vi "ColourBandPicker.vi"() -> ()   [LabVIEW 2021]
uses:
  <vilib>/userDefined/High Color/IMAQdx.ctl
  <vilib>/vision/driver/IMAQdx.llb/IMAQdx Camera Control Mode.ctl
  <vilib>/vision/driver/IMAQdx.llb/IMAQdx Acquisition Mode.ctl
  <vilib>/vision/driver/IMAQdx.llb/IMAQdx Buffer Number Mode.ctl
  <vilib>/vision/driver/NI_Vision_Acquisition_Software.lvlib
  <resource>/objmgr/imaqdx.rc
  <vilib>/vision/NI_Vision_Development_Module.lvlib
panel:
  out "Color Box":u32(colorbox)
  out "Colour Value":u32
  out "Model":string
  out "Attr":T1(array[cluster]) caption="Camera Attributes"
  out "Image":T2(plugin-control)
  in  "Stop":bool
  out "error out":errorcluster
  # "RPV Test Rig 2024"
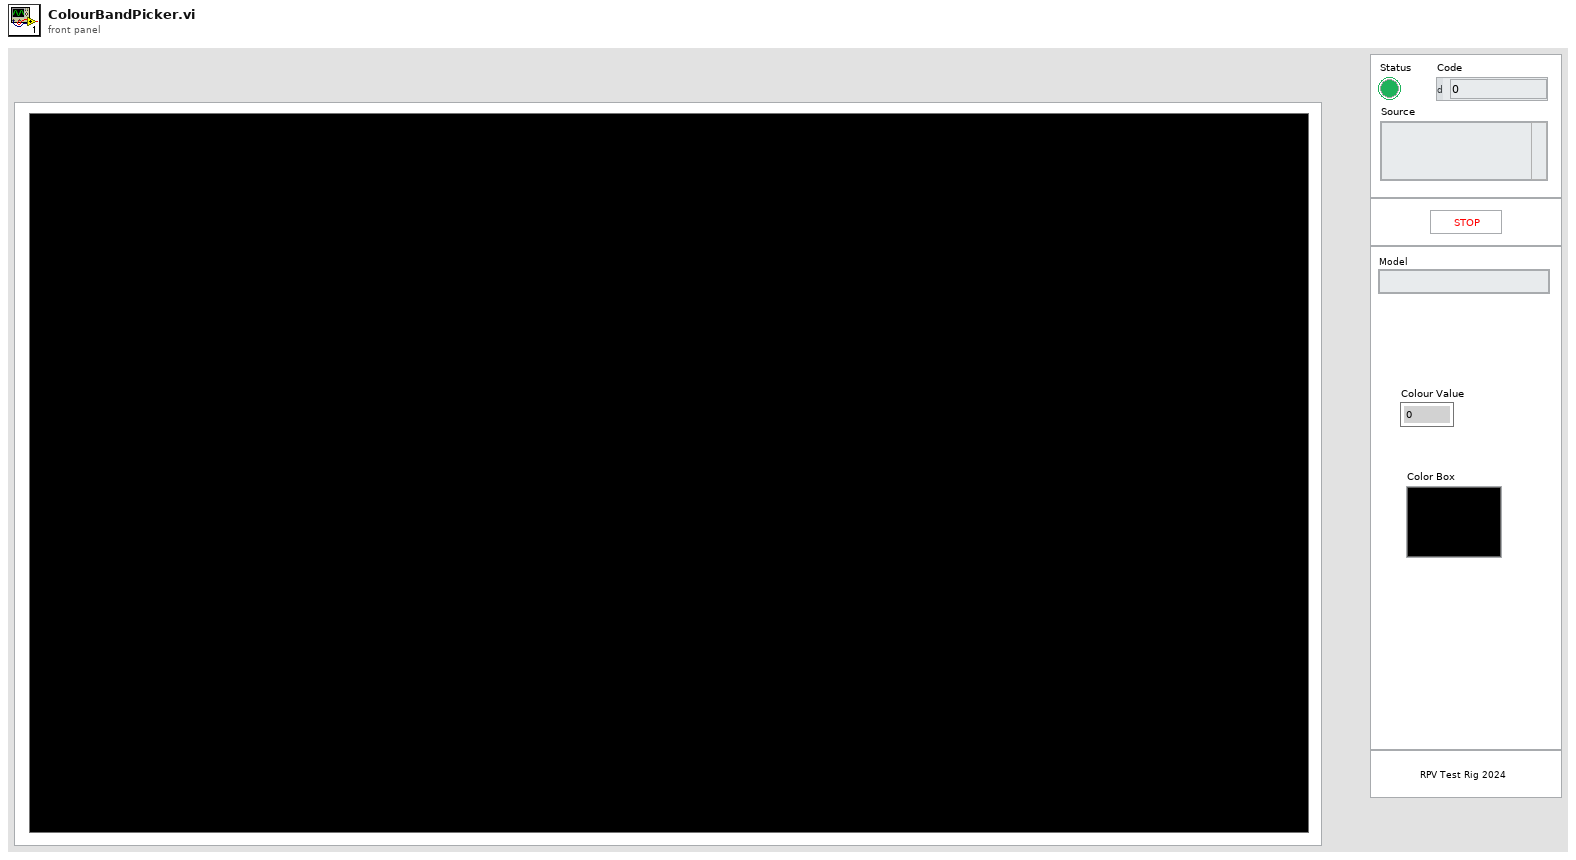
[diagram p1: front panel]
types:
  T1 = cluster{"Data Type":enum32{"U32", "I64", "DBL", "String", "Enum", "Bool", "Command"}, "Readable":bool, "Writable":bool, "Attribute Name":string}[]
  T2 = typedef "IMAQ Image.ctl" = refnum<image>
  T3 = typedef "NI_Vision_Acquisition_Software.lvlib/IMAQdx Buffer Number Mode.ctl" = enum32{"Next", "Last", "Buffer Number", "Every", "Last New"}
  T4 = typedef "NI_Vision_Acquisition_Software.lvlib/IMAQdx Acquisition Mode.ctl" = enum32{"One Shot", "Continuous"}
  T5 = typedef "NI_Vision_Acquisition_Software.lvlib/IMAQdx Camera Control Mode.ctl" = enum32{"Controller", "Listener"}
  T6 = typedef "IMAQdx.ctl" = refnum<k21>
  T7 = typedef "NI_Vision_Acquisition_Software.lvlib/IMAQdx Attribute Type.ctl" = enum32{"U32", "I64", "DBL", "String", "Enum", "Bool", "Command"}
  T8 = cluster{"Attribute Type":T7, "Readable":bool, "Writable":bool, "Attribute Name":string}[]
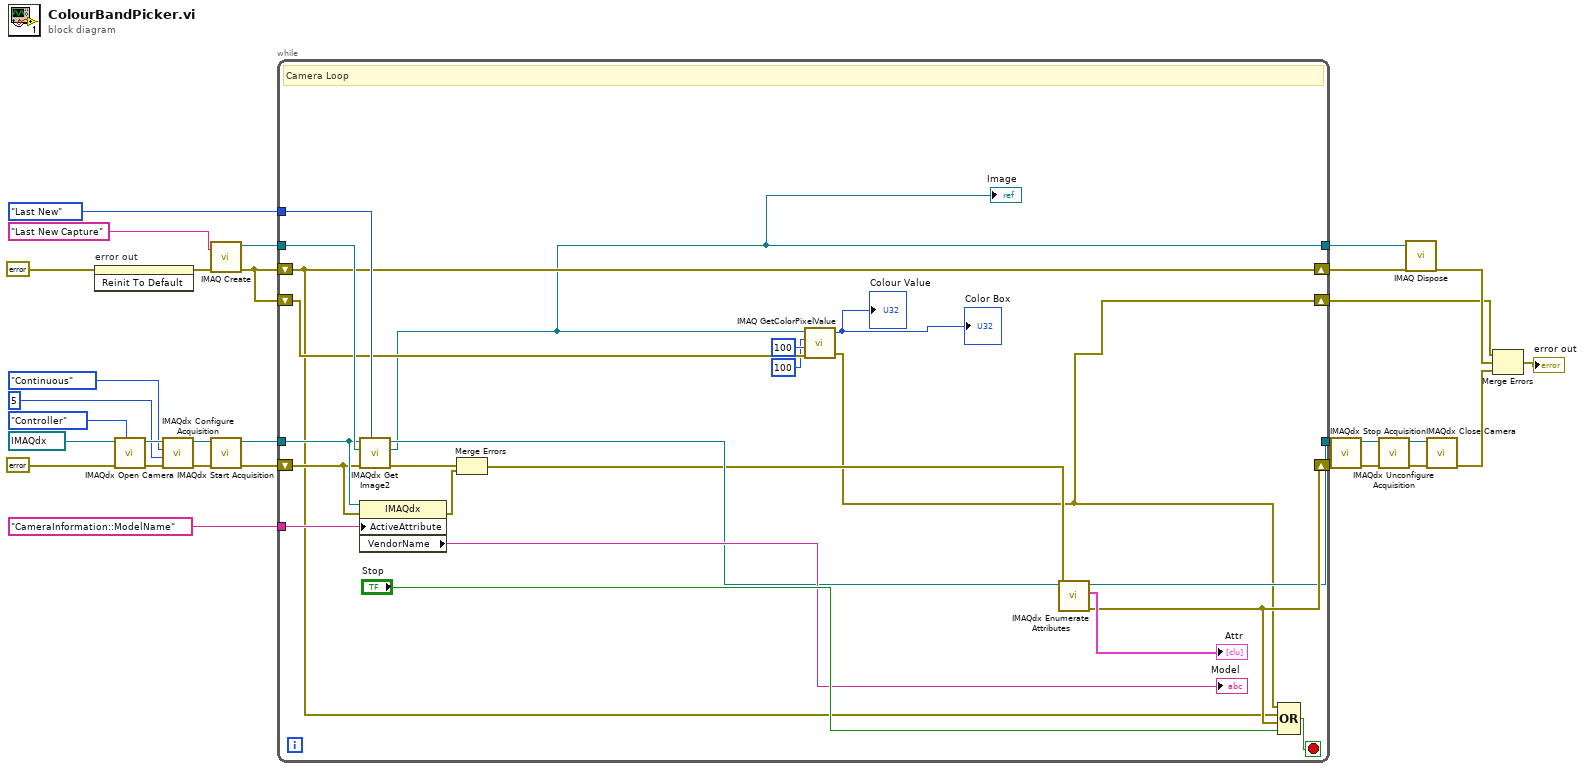
[diagram p0: block diagram]
diagram:
  n1 = invoke on="error out" class="Clust (strict)" method="Reinit To Default"(error in=errorcluster {"status"=FALSE, "code"=0, "source"=""}) -> (error out=w5:errorcluster)  [unwired: 2 in, 2 out]
  n2 = call <vilib>:"IMAQdx Open Camera.vi"("Camera Control Mode"=IMAQdx_Camera_Control_Mode."Controller", "error in"=errorcluster {"status"=FALSE, "code"=0, "source"=""}, "Session In"=T6 "cam0") -> ("error out"=w30:errorcluster, "Session Out"=w29:T6)  [unwired: 7 in]
  n3 = call <vilib>:"IMAQdx Configure Acquisition.vi"("error in"=w30, "Number of Buffers"=u32 5, "Continuous?"=IMAQdx_Acquisition_Mode."Continuous", "Session In"=w29) -> ("error out"=w24:errorcluster, "Session Out"=w23:T6)  [unwired: 6 in]
  n4 = call "IMAQ Create"("Image Name"="Last New Capture", "error in (no error)"=w5) -> ("New Image"=w12:T2, "error out"=w2:errorcluster)  [unwired: 3 in]
  n5 = call <vilib>:"IMAQdx Start Acquisition.vi"("error in"=w24, "Session In"=w23) -> ("error out"=w17:errorcluster, "Session Out"=w15:T6)  [unwired: 8 in]
  n6 = while {
    shift-right: [w45] -> w16
    shift-left: w17 -> [w42]
    tunnel: w15 -> [w43]
    tunnel: [w44] -> w14
    tunnel: IMAQdx_Buffer_Number_Mode."Last New" ("Buffer Number Mode (Next)") -> [w52]
    shift-right: [w32] -> w9
    shift-left: w2 -> [w32]
    tunnel: w12 -> [w51]
    tunnel: [w31] -> w10
    tunnel: "CameraInformation::ModelName" ("ActiveAttribute") -> [w47]
    shift-right: [w34] -> w1
    shift-left: w2 -> [w37]
    stop <- w49 stop-if-true
    # "Camera Loop"
    n7 = call <vilib>:"IMAQdx Get Image2.vi"("Buffer Number Mode (Next)"=w52, "error in"=w42, "Image In"=w51, "Session In"=w43) -> ("error out"=w41:errorcluster, "Image Out"=w31:T2, "Session Out"=w39:T6)  [unwired: 4 in, 1 out]
    "Image" <- w31
    n8 = property class="IMAQdx"(reference=w43, error in=w42, "ActiveAttribute"=w47) -> (error out=w40:errorcluster, "VendorName"=→"Model":string)  [unwired: 1 out]
    n9 = Merge Errors(w41, w40) -> (w38:errorcluster)
    n10 = call "IMAQ GetColorPixelValue"("error in (no error)"=w37, "Y Coordinate"=100, "X Coordinate"=100, "Image"=w31) -> ("error out"=w34:errorcluster, "Pixel Value (U32)"=→"Colour Value" →"Color Box":u32)  [unwired: 1 out]
    n11 = call <vilib>:"IMAQdx Enumerate Attributes.vi"("error in"=w38, "Session In"=w39) -> ("error out"=w45:errorcluster, "Attribute Information Array"=→"Attr":T8, "Session Out"=w44:T6)  [unwired: 7 in]
    n12 = Compound Arithmetic op=OR(w34, w32, w45, "Stop") -> (w49:bool)
  }
  n13 = call <vilib>:"IMAQdx Stop Acquisition.vi"("error in"=w16, "Session In"=w14) -> ("error out"=w26:errorcluster, "Session Out"=w25:T6)  [unwired: 8 in]
  n14 = call <vilib>:"IMAQdx Unconfigure Acquisition.vi"("error in"=w26, "Session In"=w25) -> ("error out"=w28:errorcluster, "Session Out"=w27:T6)  [unwired: 8 in]
  n15 = call "IMAQ Dispose"("Image"=w10, "error in (no error)"=w9) -> ("error out"=w7:errorcluster)  [unwired: 4 in]
  n16 = call <vilib>:"IMAQdx Close Camera.vi"("error in"=w28, "Session In"=w27) -> ("error out"=w6:errorcluster)  [unwired: 9 in]
  n17 = Merge Errors(w1, w7, w6) -> (→"error out":errorcluster)
